vi "FFT test.vi"() -> ()   [LabVIEW 2012, in "LightPipes.lvlib"]
uses:
  LightPipes.lvlib
  <vilib>/vision/NI_Vision_Development_Module.lvlib
panel:
  out "Output":T1(plugin-control)
  out "Input":T1(plugin-control)
  in  "File Path":path
  in  "Image Type":T2=7 items=["Grayscale (U8)", "Grayscale (I16)", "Grayscale (SGL)", "Complex (CSG)", "RGB (U32)", "HSL (U32)", "RGB (U64)", "Grayscale (U16)"]
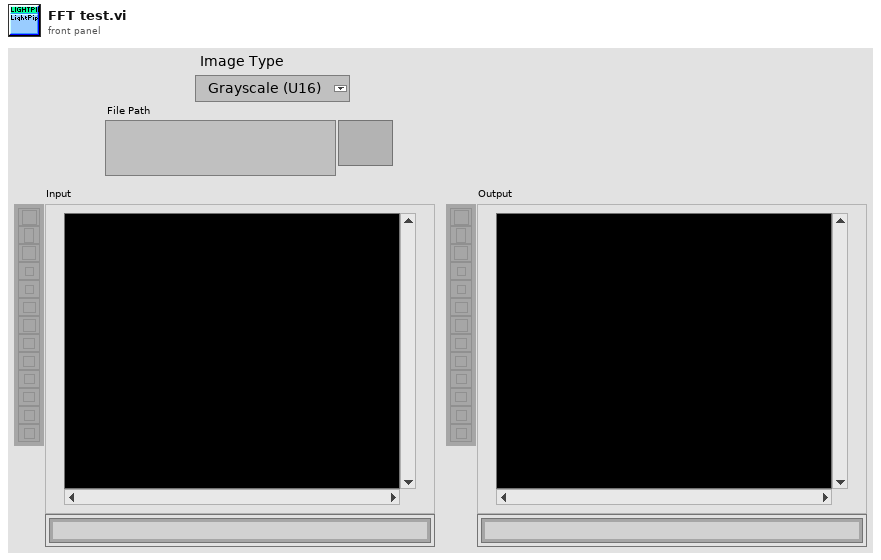
[diagram p1: front panel]
types:
  T1 = typedef "IMAQ Image.ctl" = refnum<image>
  T2 = typedef "Image Type" = u32
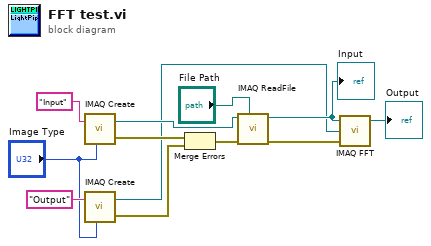
[diagram p0: block diagram]
diagram:
  n1 = call "IMAQ Create"("Image Name"="Input", "Image Type"="Image Type") -> ("New Image"=w11:T1, "error out"=w5:errorcluster)  [unwired: 3 in]
  n2 = call "IMAQ Create"("Image Name"="Output", "Image Type"="Image Type") -> ("New Image"=w1:T1, "error out"=w6:errorcluster)  [unwired: 3 in]
  n3 = Merge Errors(w5, w6) -> (w4:errorcluster)
  n4 = call "IMAQ ReadFile"("File Path"="File Path", "error in (no error)"=w4, "Image"=w11) -> ("error out"=w9:errorcluster, "Image Out"=w3:T1)  [unwired: 2 in, 5 out]
  "Input" <- w3
  n5 = call "IMAQ FFT"("error in (no error)"=w9, "Image Dst"=w1, "Image Src"=w3) -> ("Image Dst Out"=→"Output":T1)  [unwired: 1 in, 1 out]
